vi "GetInput.vi"(8 "Pads Array":T2(array[cluster]), 9 "Input Index":i32, 10 "Input Label":string, 11 "Input ID":string) -> (3 "Input":T1)   [LabVIEW 2012, in "Virtual-PGA.lvlib"]
uses:
  Virtual-PGA.lvlib
  Public/Controls/Input.ctl
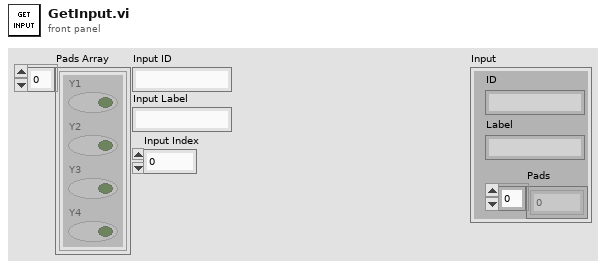
[diagram p1: front panel]
types:
  T1 = typedef "Virtual-PGA.lvlib/Input.ctl" = cluster{"ID":string, "Label":string, "Pads":u32[]}
  T2 = cluster{"Y1":bool, "Y2":bool, "Y3":bool, "Y4":bool}[]
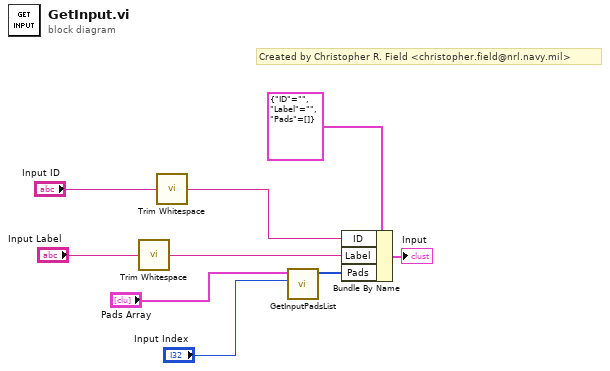
[diagram p0: block diagram]
diagram:
  # "Created by Christopher R. Field <christopher.field@nrl.navy.mil>"
  n1 = call <vilib>:"Trim Whitespace.vi"("string"="Input Label") -> ("trimmed string"=w3:string)  [unwired: 1 in]
  n2 = call <vilib>:"Trim Whitespace.vi"("string"="Input ID") -> ("trimmed string"=w1:string)  [unwired: 1 in]
  n3 = call "GetInputPadsList.vi"("Input Index"="Input Index", "Pads Array"="Pads Array") -> ("Input Pads List"=w8:u32[])  [unwired: 9 in]
  n4 = Bundle By Name(cluster=T1 {"ID"="", "Label"="", "Pads"=[]} ("Input"), "ID"=w1, "Label"=w3, "Pads"=w8) -> (→"Input":T1)
